vi "ex_setTdmProperty_DBL.vi"(4 "Strings":string[](array[string]), 5 "Values":i32[](array[numeric]), 6 "Value":dbl, 7 "Name":string) -> (3 "output cluster":T1)   [LabVIEW 2017]
uses:
  <vilib>/express/express shared/ExFile.llb/ex_TdmProperty.ctl
  <vilib>/express/express shared/ex_EditUserDefinedProperties/usiDataType.ctl
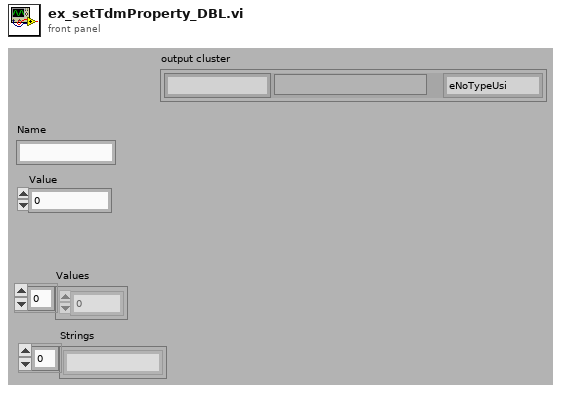
[diagram p1: front panel]
types:
  T1 = typedef "ex_TdmProperty.ctl" = cluster{"Name":string, "Type":T2, "Value":variant}
  T2 = typedef "usiDataType.ctl" = enum16{"eNoTypeUsi", "eInt8Usi", "eInt16Usi", "eInt32Usi", "eInt64Usi", "eUInt8Usi", "eUInt16Usi", "eUInt32Usi", "eUInt64Usi", "eFloat32Usi", "eFloat64Usi", "- 0", "- 1", "- 2", "- 3", "- 4", "- 5", "- 6", "- 7", "- 8", "- 9", "eString8Usi", "eString16Usi", "eStringUsi", "eEnumUsi", "- 10", "- 11", "- 12", "- 13", "- 14", "eTimeUsi", "- 15", "- 16", "- 17", "- 18", "- 19", "- 20", "- 21", "- 22", "- 23", "eInstanceUsi", "eStoreUsi"}
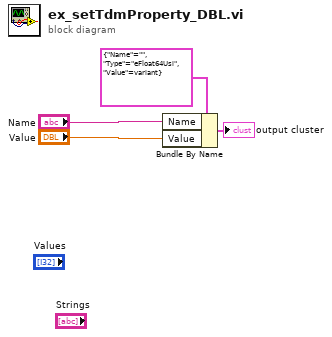
[diagram p0: block diagram]
diagram:
  n1 = Bundle By Name(cluster=T1 {"Name"="", "Type"=enum."eFloat64Usi", "Value"=variant} ("TDM Property"), "Name"="Name", "Value"="Value") -> (→"output cluster":T1)
